vi "Unlock focus.vi"(8 "error in":errorcluster, 11 "VISA resource in":refnum<visa-resource-name>) -> (0 "error out":errorcluster, 3 "VISA resource out":refnum<visa-resource-name>)   [LabVIEW 2018]
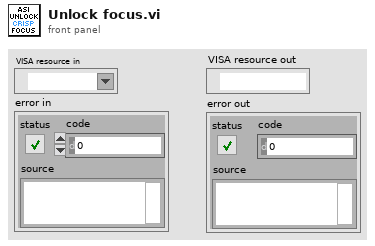
[diagram p1: front panel]
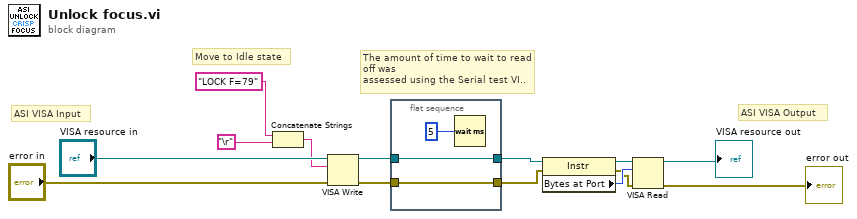
[diagram p0: block diagram]
diagram:
  # "Move to Idle state"
  # "ASI VISA Output"
  # "ASI VISA Input"
  # "The amount of time to wait to read off was \nassessed using the Serial test VI.."
  n1 = Concatenate Strings("LOCK F=79" ("write buffer"), "\r") -> (w11:string)
  n2 = VISA Write(VISA resource name="VISA resource in", write buffer=w11, error in (no error)="error in") -> (VISA resource name out=w7:refnum<visa-resource-name>, error out=w8:errorcluster)  [unwired: 1 out]
  n3 = flat-sequence {
    tunnel: [w17] -> w10
    tunnel: w7 -> [w17]
    tunnel: [w15] -> w9
    tunnel: w8 -> [w15]
    frame #0 {
      n4 = Wait (ms)(milliseconds to wait=u32 5) -> ()  [unwired: 1 out]
    }
  }
  n5 = property class="Instr"(reference=w10, error in=w9) -> (reference out=w6:refnum<visa-resource-name>, error out=w4:errorcluster, "Bytes at Port"=w5:u32)
  n6 = VISA Read(VISA resource name=w6, byte count=w5, error in (no error)=w4) -> (VISA resource name out=→"VISA resource out":refnum<visa-resource-name>, error out=→"error out":errorcluster)  [unwired: 2 out]
